vi "AnyBuilderBeginRepeatedNestedMessageElement.vi"(8 "error in (no error)":errorcluster, 11 "gRPCid in":T1) -> (0 "error out":errorcluster, 2 "Nested Element ID":T1, 3 "gRPCid":T1)   [LabVIEW 2019, in "TestDataMarshal.lvlib" / "gprc-lvsupport.lvlib"]
uses:
  gprc-lvsupport.lvlib
  typeDefs/grpcId.ctl
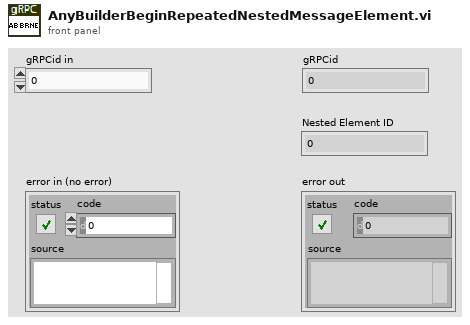
[diagram p1: front panel]
types:
  T1 = typedef "TestDataMarshal.lvlib/gprc-lvsupport.lvlib/grpcId.ctl" = u64
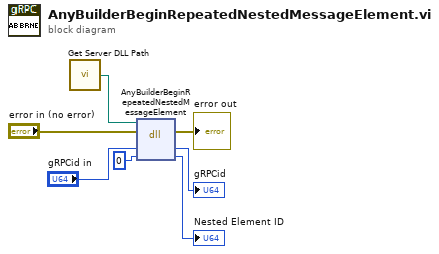
[diagram p0: block diagram]
diagram:
  n1 = call "Get Server DLL Path.vi"() -> ("Server dll path"=w3:path)
  n2 = dll-call lib="?" fn="AnyBuilderBeginRepeatedNestedMessageElement"(path in=w3, error in="error in (no error)", "builderId"="gRPCid in", "nestedId"=u64 0) -> (error out=→"error out":errorcluster, "builderId"=→"gRPCid":u64, "nestedId"=→"Nested Element ID":u64)  [unwired: 2 in, 1 out]
